vi "file operation.vi"(8 "error in":errorcluster, 11 "File in":refnum<class "File.lvclass">) -> (0 "error out":errorcluster, 3 "File out":refnum<class "File.lvclass">)   [LabVIEW 2023, in "File Classes.lvlib" / "File.lvclass"]
uses:
  File.lvclass
  File.lvclass/File.ctl
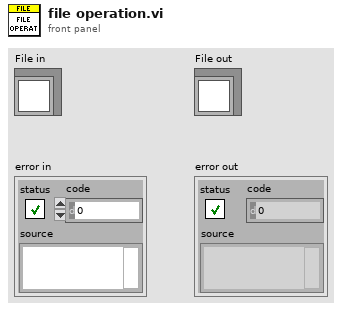
[diagram p1: front panel]
types:
  T1 = typedef "File Classes.lvlib/file operation enum.ctl" = enum16{"Copying", "Moving", "Deleting", "Skiped", "Renaming"}
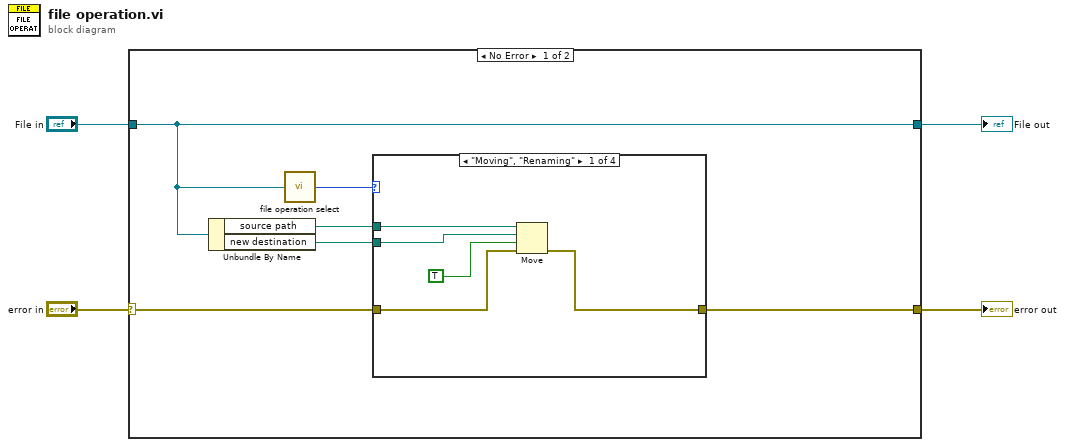
[diagram p0: block diagram]
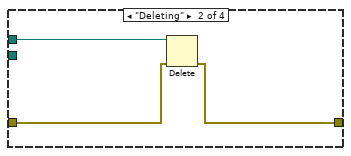
[diagram p2: hidden frame]
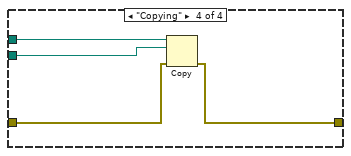
[diagram p4: hidden frame]
diagram:
  n1 = case shown="No Error" "error in" {
    selector: "error in" -> [w8 w25]
    tunnel: [w7 w25] -> w3
    tunnel: [w6 w24] -> w1
    tunnel: "File in" -> [w6 w24]
    frame No Error {
      n2 = Unbundle By Name(w6) -> ("source path"=w10:path, "new destination"=w9:path)
      n3 = call "file operation select.vi"("File in"=w6) -> ("Operation"=w5:T1)
      n4 = case shown="\"Moving\", \"Renaming\"" w5 {
        tunnel: w10 -> [w13 w18 _ w23]
        tunnel: w9 -> [w12 _ _ w20]
        tunnel: w8 -> [w15 w17 w19 w22]
        tunnel: [w14 w16 w19 w21] -> w7
        frame "Moving", "Renaming" {
          n5 = Move(source path=w13, error in=w15, 9:TRUE ("overwrite (F)"), 10:w12) -> (error out=w14:errorcluster)  [unwired: 1 in, 2 out]
        }
        frame "Deleting" {
          n6 = Delete(path (use dialog)=w18, error in=w17) -> (error out=w16:errorcluster)  [unwired: 3 in, 2 out]
        }
        frame "Skiped" {
        }
        frame "Copying" {
          n7 = Copy(8:w22, 10:w20, 11:w23) -> (0:w21:errorcluster)  [unwired: 2 in, 2 out]
        }
      }
    }
    frame Error {
    }
  }
  "error out" <- w3
  "File out" <- w1
